vi "FlatToRichcif_template_GetStatisticsRequest.vi"(5 "OutputClusterType":T1, 11 "InputCluster":T2) -> (3 "OutputCluster":T1)   [LabVIEW 2021, in "Template_client.lvlib"]
uses:
  cif_template_GetStatisticsRequest_Flat.ctl
  cif_template_GetStatisticsRequest.ctl
  Template_client.lvlib
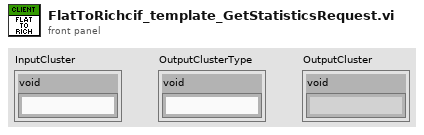
[diagram p1: front panel]
types:
  T1 = typedef "Template_client.lvlib/cif_template_GetStatisticsRequest.ctl" = cluster{"void":string}
  T2 = typedef "Template_client.lvlib/cif_template_GetStatisticsRequest_Flat.ctl" = cluster{"void":string}
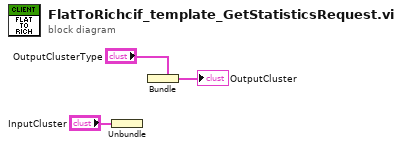
[diagram p0: block diagram]
diagram:
  n1 = Unbundle "Unbundle"("InputCluster") -> ()  [unwired: 1 out]
  n2 = Bundle "Bundle"(cluster="OutputClusterType") -> (→"OutputCluster":T1)  [unwired: 1 in]
